vi "read analog in settings json.vi"(10 "AI channel type":T1 {"units" items=["Volts"=10348, "From TEDS"=12516, "From Custom Scale"=10065]}, 11 "appended path":path) -> (2 "AI channel settings out":T1 {"units" items=["Volts"=10348, "From TEDS"=12516, "From Custom Scale"=10065]})   [LabVIEW 2018]
uses:
  DAQ_inputs/AI channel settings.ctl
  <vilib>/addons/_JKI.lib/Serialization/JSON/JKI JSON Serialization.lvlib
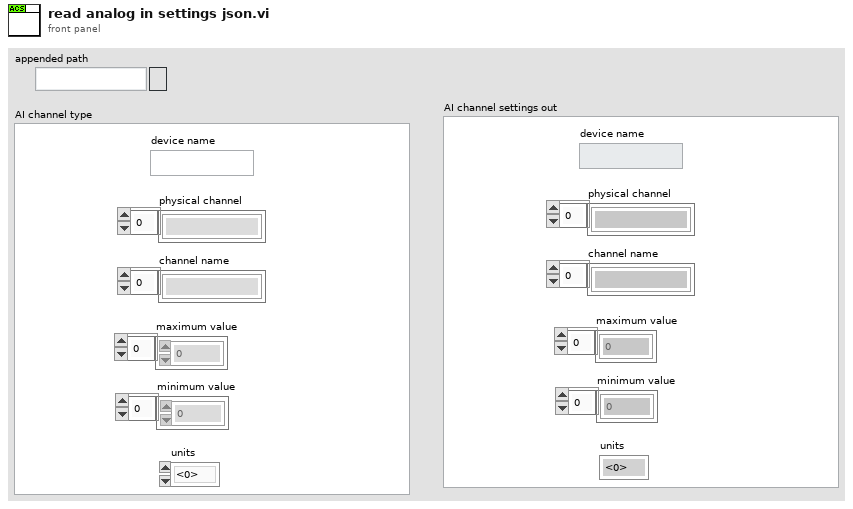
[diagram p1: front panel]
types:
  T1 = typedef "AI channel settings.ctl" = cluster{"device name":string, "physical channel":string[], "channel name":string[], "maximum value":dbl[], "minimum value":dbl[], "units":i32}
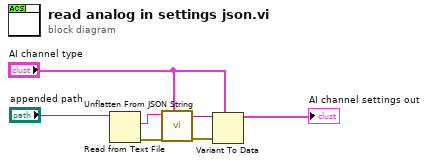
[diagram p0: block diagram]
diagram:
  n1 = Read from Text File(file (use dialog)="appended path") -> (text=w1:string, error out=w2:errorcluster)  [unwired: 3 in, 2 out]
  n2 = call <vilib>:"Unflatten From JSON String.vi"("Type and Defaults"="AI channel type", "error in (no error)"=w2, "JSON String"=w1) -> ("error out"=w3:errorcluster, "Variant"=w4:variant)  [unwired: 7 in]
  n3 = Variant To Data(error in=w3, type="AI channel type", Variant=w4) -> (data=→"AI channel settings out":T1)  [unwired: 1 out]
